vi "Initialize and Sort Key Values.vi"() -> (8 "refnum":T1, 11 "Preferences":string[][](array[string]))   [LabVIEW 2015]
uses:
  <vilib>/Utility/config.llb/Config Data RefNum.ctl
  <vilib>/Rock Robotics/Network Tables/NT Read String.vi
  <vilib>/Utility/config.llb/Read Key (String).vi
  <vilib>/Utility/config.llb/NI_LVConfig.lvlib
panel:
  out "error out":errorcluster
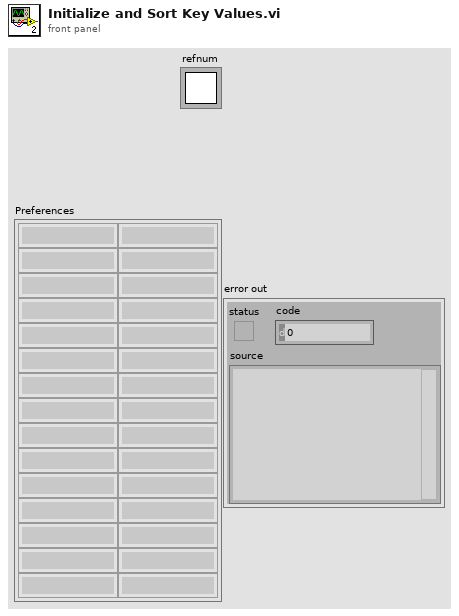
[diagram p1: front panel]
types:
  T1 = typedef "NI_LVConfig.lvlib/Config Data RefNum.ctl" = refnum<k1>
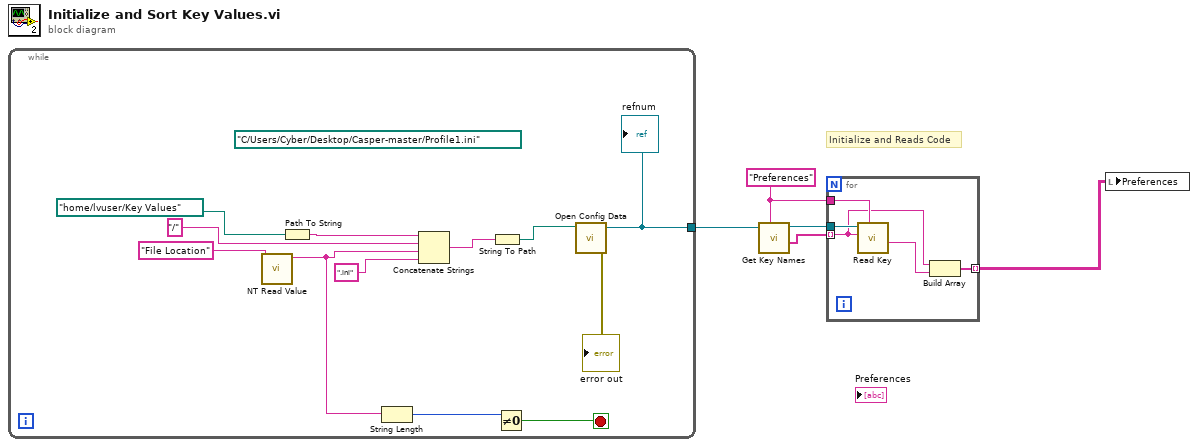
[diagram p0: block diagram]
diagram:
  w4 = "Preferences" ("section")
  # "Initialize and Reads Code"
  n1 = while {
    tunnel: [w6] -> w1
    stop <- w8 stop-if-true
    (unwired) path "C:/Users/Cyber/Desktop/Casper-master/Profile1.ini" ("path")
    n2 = call-poly <vilib>:"NT Read Value.vi"("Name"="File Location") -> ("String"=w10:string)  [unwired: 9 in, 1 out]
    n3 = Path To String(path=path "/home/lvuser/Key Values" ("configuration file path")) -> (string=w17:string)
    n4 = String Length(string=w10) -> (length=w9:i32)
    n5 = Concatenate Strings(w17, "/" ("string"), w10, ".ini" ("string")) -> (w16:string)
    n6 = String To Path(string=w16) -> (path=w7:path)
    n7 = Not Equal To 0?(x=w9) -> (x != 0?=w8:bool)
    n8 = call <vilib>:"Open Config Data.vi"("configuration file path"=w7) -> ("error out"=→"error out":errorcluster, "refnum"=w6:T1)  [unwired: 8 in, 1 out]
    "refnum" <- w6
  }
  n9 = call <vilib>:"Get Key Names.vi"("section"=w4, "refnum"=w1) -> ("key names"=w5:string[], "refnum out"=w3:T1)  [unwired: 6 in, 2 out]
  n10 = for {
    tunnel: w5 -> [w20] mode=indexing
    tunnel: w3 -> [w22]
    tunnel: w4 -> [w21]
    tunnel: [w18] -> w2 mode=indexing
    n11 = call-poly <vilib>:"Read Key.vi"("section"=w21, "key"=w20, "refnum"=w22) -> ("value"=w19:string)  [unwired: 5 in, 3 out]
    n12 = Build Array(w20, w19) -> (w18:string[])
  }
  n13 = local write "Preferences"(w2) -> ()
